vi "Measure vs B2D.vi"() -> ()   [LabVIEW 2009]
doc: "This VI is an example operator panel.\n\nThe VI contains a table for the field values that may be configured manually, or loaded by checking the \"Prompt for File\" box. The data file should contain 3 columns of data, with each column delimited by a tab character.\n\nBefore the VI is executed, set the desired field units and coordinate system. Once the VI is started, follow the directions in the STATUS indicator to operate. Once a field value is achieved, it will be held indefinitely with no user intervention.\n\nThe present field is displayed in the selected units and coordinate system. The present field is queried once per second.\n\nIf a field point is specified that is outside the limits for the magnet, the VI will abort execution."
uses:
  <vilib>/Utility/file.llb/Read From Spreadsheet File (DBL).vi
panel:
  in  "X Axis":enum16{"B", "phi"}(ring)
  in  "Y Axis":T1(ring)=enum."LI 1 Vx"
  out "measured data":dbl[][](array[numeric])
  out "XY Graph":T2(graph)
  in  "Notes:":string caption="Notizen:"
  out "Messfile Refnum":refnum<file>
  in  "Measurement File":path=path "D:/UserData/Matthias/Test/test.txt"
  in  "Sample name:":string
  in  "HP 1":bool
  in  "GPIB HP":string="8"
  in  "LI 4":bool
  in  "GPIB L 4":string="8"
  in  "LI 3":bool
  in  "GPIB L 3":string="8"
  in  "LI 2":bool
  in  "GPIB L 2":string="8"
  in  "LI 1":bool=TRUE
  in  "GPIB L 1":string="8"
  out "Number of lines":i32=2
  in  "Operation":u16(ring) items=["Stepwise", "Continous"]
  out "Ramp Rate along Vector (T/min)":dbl=0.17799999999999996 format="%.3f"
  out "Current Ramp Rate Z (T/min)":dbl=0.17799999911017794 format="%.3f"
  out "Current Ramp Rate Y (T/min)":dbl=1.7798220089008895e-05 format="%.3f"
  in  "User defined Ramp Rate (T/min)":bool=TRUE
  in  "User defined Ramp Rate (T/min)":dbl=0.178 format="%.3f"
  in  "Z-Axis Communications Config":T3={"GPIB address"=22, "GPIB bus"=1, "connection ID"=refnum, "IP"="111.111.111.1", "Active Comm Interface"=0, "Serial Port"="", "Programmer Type"=0} {"Programmer Type" items=["Model 430", "Model 420"]; "Active Comm Interface" items=["TCP/IP (Model 430 Only)", "RS232", "IEEE488"]}
  in  "Max Ramp Rate - Y Axis (A/s)":dbl=0.065 format="%.3f"
  in  "Max Ramp Rate - Z Axis (A/s)":dbl=0.203 format="%.3f"
  in  "Magnitude Limit (kG)":dbl=45.1 format="%.3f"
  in  "Y-Axis Communications Config":T3={"GPIB address"=22, "GPIB bus"=1, "connection ID"=refnum, "IP"="111.111.111.2", "Active Comm Interface"=0, "Serial Port"="", "Programmer Type"=0} {"Programmer Type" items=["Model 430", "Model 420"]; "Active Comm Interface" items=["TCP/IP (Model 430 Only)", "RS232", "IEEE488"]}
  out "Cartesian Display (T)":T4={"Y-Axis Field (T)"=-0.0, "Z-Axis Field (T)"=1e-05} {"Z-Axis Field (T)" format="%.3f"; "Y-Axis Field (T)" format="%.3f"}
  in  "Starting index":i32
  in  "Normal color":u32(colorbox)=11711154
  in  "Highlight color":u32(colorbox)=16711680
  out "?":string="American Magnetics, Inc."
  in  "Prompt for File?":bool
  out "Continue Execution?":bool=TRUE
  out "error out":T5
  in  "error in":T5
  out "STATUS":string="Holding at current vector. Set Ramping Mode to NEXT VECTOR to continue."
  in  "Ramping Control":u16(ring)=2 items=["NEXT VECTOR", "RAMPING", "HOLDING", "PAUSE", "ZERO"]
  out "Cartesian Display (kG)":T6 {"Z-Axis Field (kG)" format="%.3f"; "Y-Axis Field (kG)" format="%.3f"}
  in  "Field Values":string[][](table)=[["0", "0.1"], ["0", "0"]]
  out "Switch Heaters":bool=TRUE
  out "Polar Display (T)":T7={"q (degrees)"=90.0, "Field Magnitude (T)"=2e-05} {"Field Magnitude (T)" format="%.3f"; "q (degrees)" format="%.3f"}
  out "Polar Display (kG)":T8 {"Field Magnitude (kG)" format="%.3f"; "q (degrees)" format="%.3f"}
  in  "Coordinate System":u16(ring) items=["Cartesian", "Polar"]
  in  "Magnetic Field Units":u16(ring)=1 items=["kG", "Tesla"]
  # "Measurement Display"
  # "Measurement Settings"
  # "Magnet Settings"
  # "Devices"
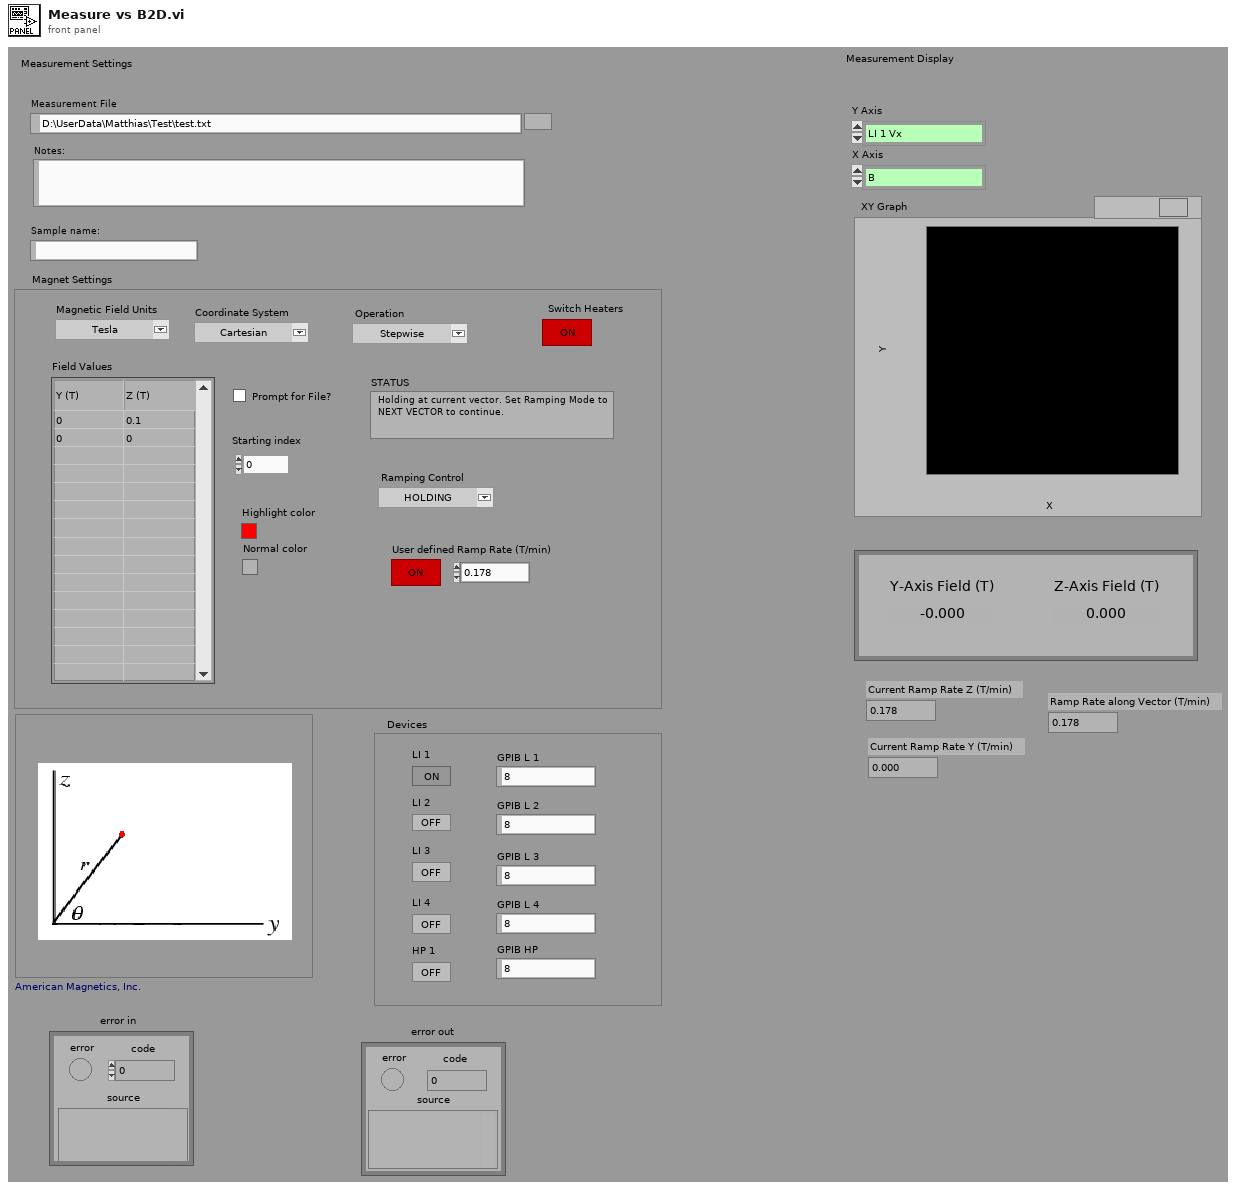
[diagram p1: front panel]
types:
  T1 = enum16{"B", "phi", "LI 1 Vx", "LI 1 phase", "LI 2 Vx", "LI 2 phase", "LI 3 Vx", "LI 3 phase", "LI 4 Vx", "LI 4 phase", "HP (V)"}
  T2 = cluster{"measured data":dbl[], "measured data":dbl[]}
  T3 = cluster{"GPIB address":i16, "GPIB bus":i16, "connection ID":refnum<k5>, "IP":string, "Active Comm Interface":u16, "Serial Port":refnum<visa-resource-name>, "Programmer Type":u16}
  T4 = cluster{"Y-Axis Field (T)":dbl, "Z-Axis Field (T)":dbl}
  T5 = cluster{"error":bool, "code":i32, "source":string}
  T6 = cluster{"Y-Axis Field (kG)":dbl, "Z-Axis Field (kG)":dbl}
  T7 = cluster{"q (degrees)":dbl, "Field Magnitude (T)":dbl}
  T8 = cluster{"q (degrees)":dbl, "Field Magnitude (kG)":dbl}
  T9 = enum16{"", "RAMPING", "HOLDING", "PAUSED", "MANUAL UP", "MANUAL DOWN", "ZEROING CURRENT", "QUENCH DETECTED", "HEATING SWITCH"}
  T10 = enum16{"", "RAMPING", "HOLDING", "PAUSED", "MANUAL UP", "MANUAL DOWN", "ZEROING CURRENT", "QUENCH DETECTED", "HEATING SWITCH", "AT ZER0", "COOLING SWITCH"}
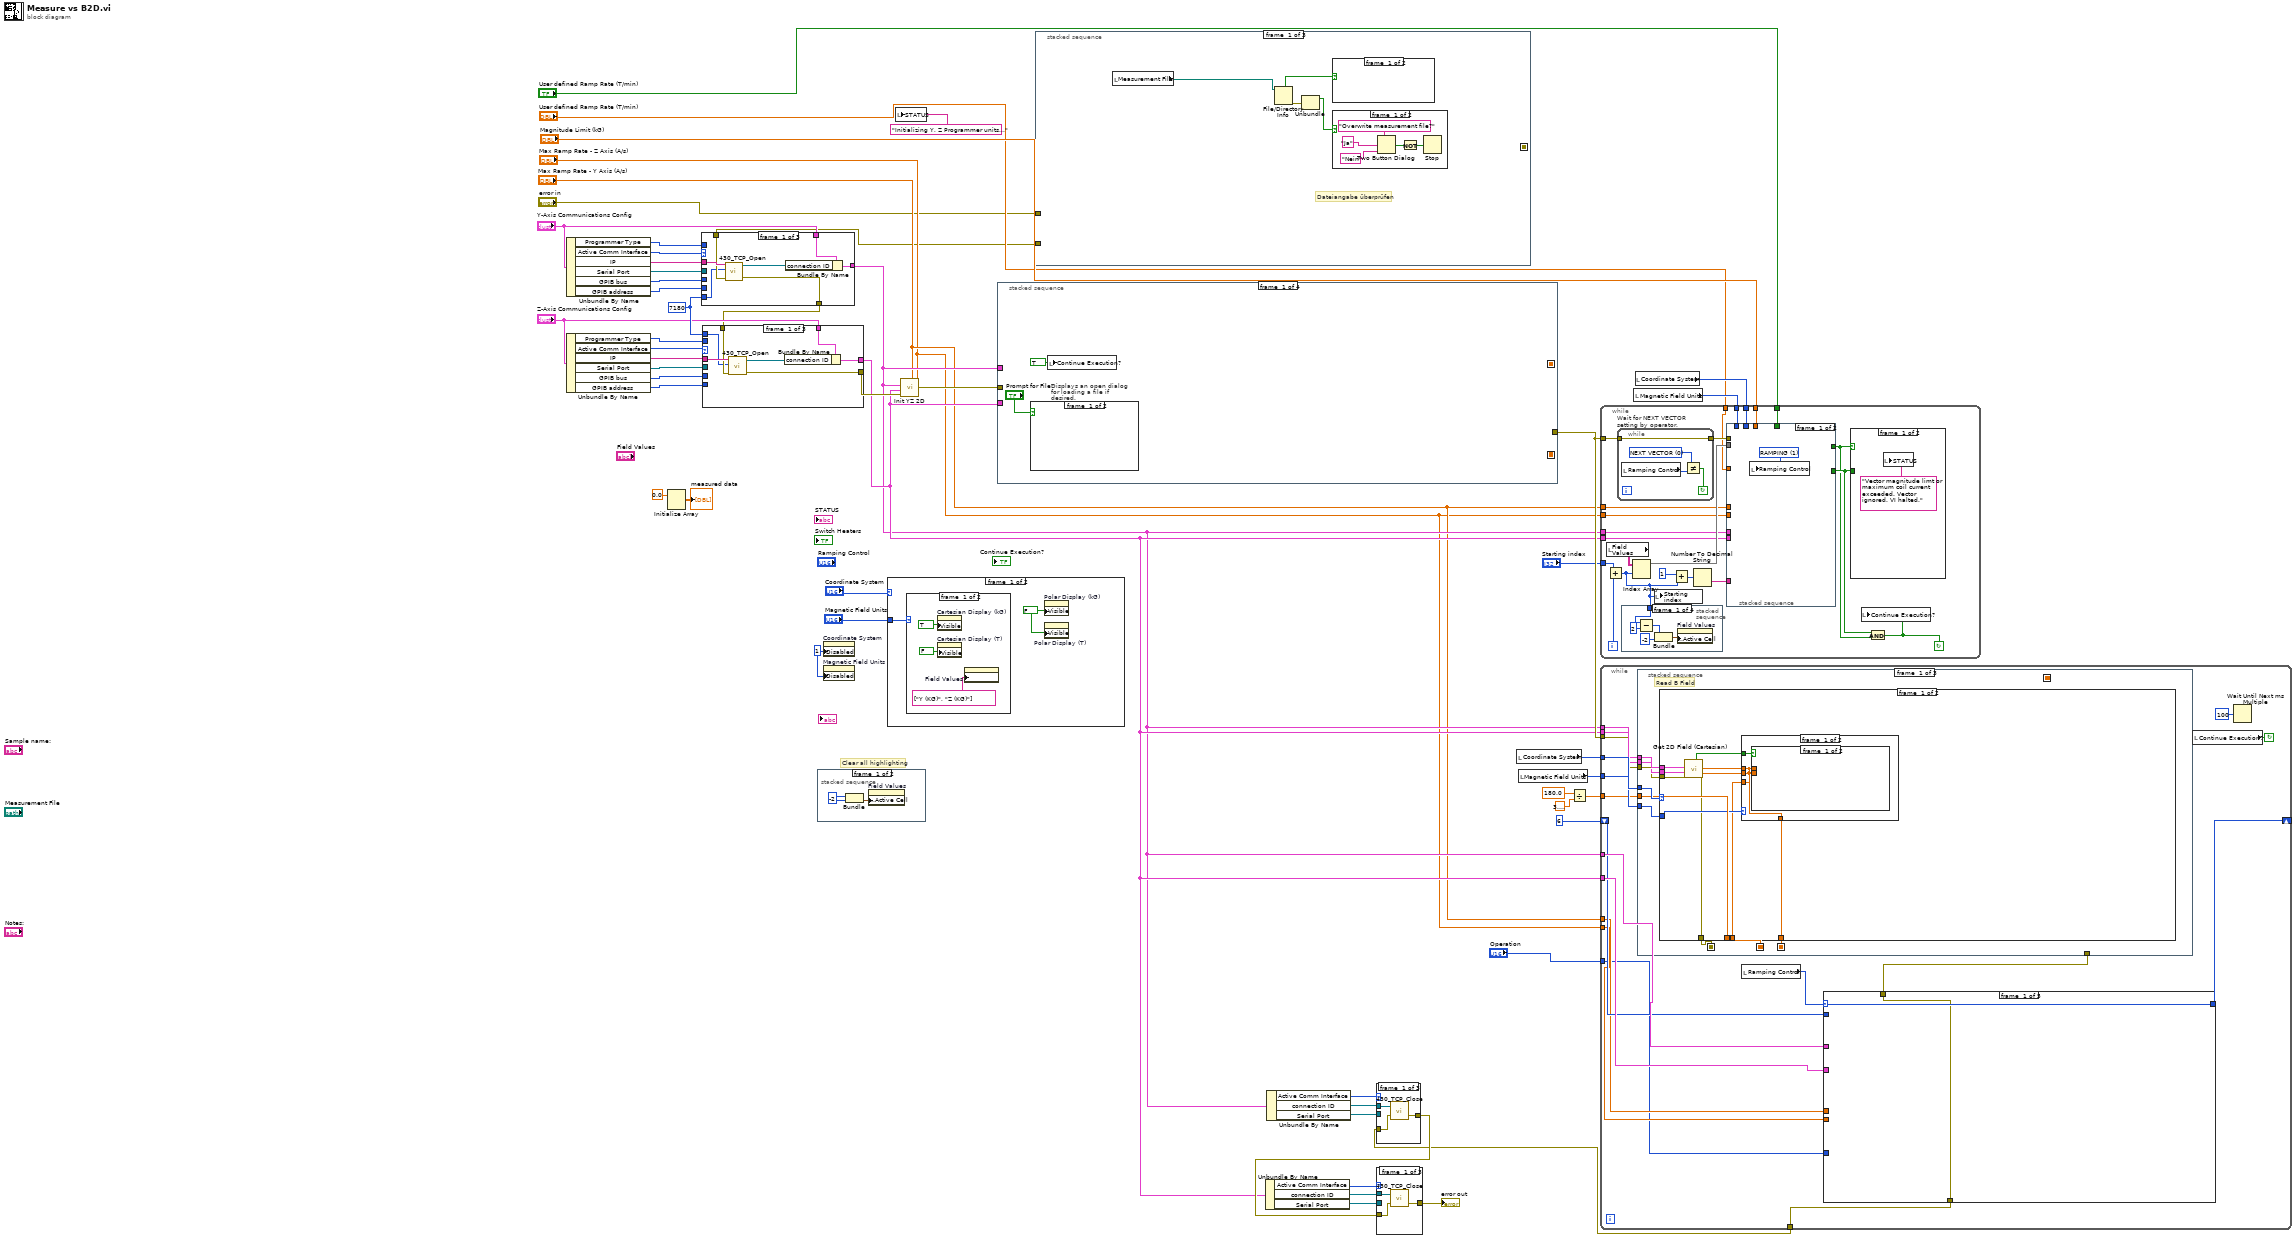
[diagram p0: block diagram]
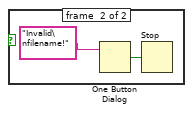
[diagram p3: hidden frame]
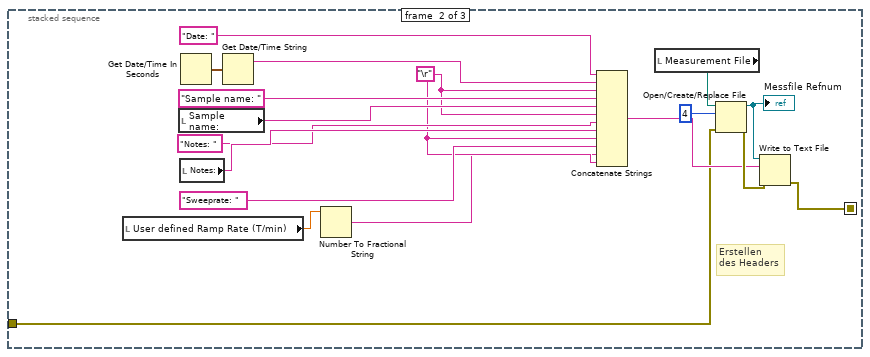
[diagram p4: hidden frame]
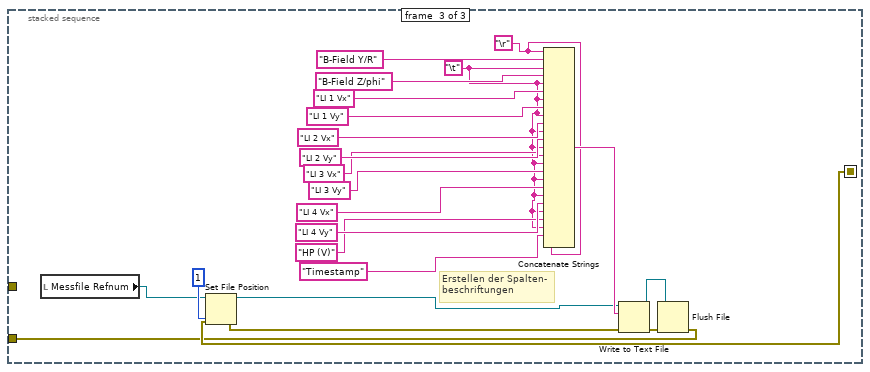
[diagram p5: hidden frame]
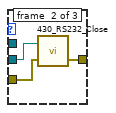
[diagram p6: hidden frame]
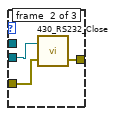
[diagram p8: hidden frame]
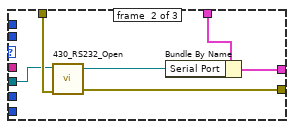
[diagram p10: hidden frame]
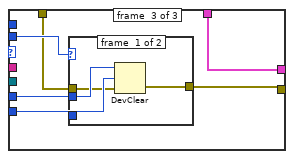
[diagram p11: hidden frame]
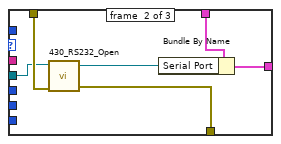
[diagram p13: hidden frame]
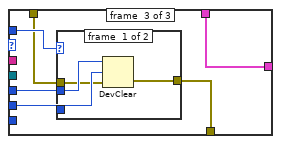
[diagram p14: hidden frame]
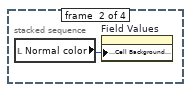
[diagram p16: hidden frame]
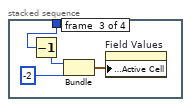
[diagram p17: hidden frame]
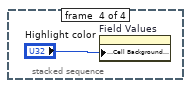
[diagram p18: hidden frame]
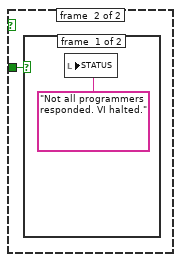
[diagram p19: hidden frame]
diagram:
  w38 = 7180 ("TCP Port")
  w51 = u8 1 ("Write Attribute")
  # "Clear all highlighting"
  n1 = Unbundle By Name("Z-Axis Communications Config") -> ("Programmer Type"=w14:u16, "Active Comm Interface"=w37:u16, "IP"=w34:string, "Serial Port"=w33:refnum<visa-resource-name>, "GPIB bus"=w13:i16, "GPIB address"=w12:i16)
  n2 = Unbundle By Name("Y-Axis Communications Config") -> ("Programmer Type"=w8:u16, "Active Comm Interface"=w36:u16, "IP"=w35:string, "Serial Port"=w32:refnum<visa-resource-name>, "GPIB bus"=w9:i16, "GPIB address"=w10:i16)
  n3 = Initialize Array(0.0 ("element")) -> (→"measured data":dbl[][])  [unwired: 2 in]
  n4 = stacked-sequence {
    frame #0 {
      w54 = -2
      n5 = Bundle(w54, w54) -> (w55:cluster{i32, i32})  [unwired: 1 in]
      n6 = property on="Field Values" class="Tbl (strict)"("Active Cell:Active Cell"=w55) -> ()  [unwired: 2 in, 2 out]
    }
    frame #1 {
      n7 = property on="Field Values" class="Tbl (strict)"("Active Cell:Cell Background Color"="Normal color") -> ()  [unwired: 2 in, 2 out]
    }
  }
  n8 = property on="Coordinate System" class="Ring (strict)"("Disabled"=w51) -> ()  [unwired: 2 in, 2 out]
  n9 = property on="Magnetic Field Units" class="Ring (strict)"("Disabled"=w51) -> ()  [unwired: 2 in, 2 out]
  n10 = case shown="1" "Coordinate System" {
    tunnel: "Magnetic Field Units" -> [w58 w66]
    frame #0 {
      w57 = FALSE ("Write Attribute")
      (unwired) FALSE ("Write Attribute")
      (unwired) TRUE ("Write Attribute")
      n11 = case shown="0, Default" w58 {
        frame #0 {
          n12 = property on="Cartesian Display (kG)" class="Cluster (strict)"("Visible"=TRUE ("Write Attribute")) -> ()  [unwired: 2 in, 2 out]
          n13 = property on="Cartesian Display (T)" class="Cluster (strict)"("Visible"=FALSE ("Write Attribute")) -> ()  [unwired: 2 in, 2 out]
          n14 = property on="Field Values" class="Tbl (strict)"("Column Header Strings[]"=string[] ["Y (KG)", "Z (KG)"] ("Write Attribute")) -> ()  [unwired: 2 in, 2 out]
        }
        frame #1 {
          n15 = property on="Cartesian Display (kG)" class="Cluster (strict)"("Visible"=FALSE ("Write Attribute")) -> ()  [unwired: 2 in, 2 out]
          n16 = property on="Cartesian Display (T)" class="Cluster (strict)"("Visible"=TRUE ("Write Attribute")) -> ()  [unwired: 2 in, 2 out]
          n17 = property on="Field Values" class="Tbl (strict)"("Column Header Strings[]"=string[] ["Y (T)", "Z (T)"] ("Write Attribute")) -> ()  [unwired: 2 in, 2 out]
        }
      }
      n18 = property on="Polar Display (kG)" class="Clust (strict)"("Visible"=w57) -> ()  [unwired: 2 in, 2 out]
      n19 = property on="Polar Display (T)" class="Clust (strict)"("Visible"=w57) -> ()  [unwired: 2 in, 2 out]
    }
    frame #1 {
      (unwired) FALSE ("Write Attribute")
      (unwired) TRUE ("Write Attribute")
      w65 = FALSE ("Write Attribute")
      n20 = case shown="1" w66 {
        frame #0 {
          n21 = property on="Polar Display (kG)" class="Clust (strict)"("Visible"=TRUE ("Write Attribute")) -> ()  [unwired: 2 in, 2 out]
          n22 = property on="Polar Display (T)" class="Clust (strict)"("Visible"=FALSE ("Write Attribute")) -> ()  [unwired: 2 in, 2 out]
          n23 = property on="Field Values" class="Tbl (strict)"("Column Header Strings[]"=string[] ["Mag. r (KG)", "Theta (deg)"] ("Write Attribute")) -> ()  [unwired: 2 in, 2 out]
        }
        frame #1 {
          n24 = property on="Polar Display (kG)" class="Clust (strict)"("Visible"=FALSE ("Write Attribute")) -> ()  [unwired: 2 in, 2 out]
          n25 = property on="Polar Display (T)" class="Clust (strict)"("Visible"=TRUE ("Write Attribute")) -> ()  [unwired: 2 in, 2 out]
          n26 = property on="Field Values" class="Tbl (strict)"("Column Header Strings[]"=string[] ["Mag. r (T)", "Theta (deg)"] ("Write Attribute")) -> ()  [unwired: 2 in, 2 out]
        }
      }
      n27 = property on="Cartesian Display (kG)" class="Cluster (strict)"("Visible"=w65) -> ()  [unwired: 2 in, 2 out]
      n28 = property on="Cartesian Display (T)" class="Cluster (strict)"("Visible"=w65) -> ()  [unwired: 2 in, 2 out]
    }
  }
  n29 = local write "STATUS"("Initializing Y, Z Programmer units..." ("STATUS")) -> ()
  n30 = stacked-sequence {
    seq-local: [_ w84 _] -> [_ _ w103]
    tunnel: "error in" -> [_ w85 _]
    tunnel: [_ _ w102] -> w3
    frame #0 {
      # "Dateiangabe überprüfen"
      n31 = local read "Measurement File"() -> (w76:path)
      n32 = File/Directory Info(path=w76) -> (directory=w74:bool, error out=w75:errorcluster)  [unwired: 1 in, 5 out]
      n33 = Unbundle(w75) -> ("status"=w73:bool)  [unwired: 2 out]
      n34 = case shown="False" w74 {
        frame #0 {
        }
        frame #1 {
          n35 = One Button Dialog(message="Invalid\nfilename!") -> (true=w82:bool)  [unwired: 1 in]
          n36 = Stop(stop? (T)=w82) -> ()
        }
      }
      n37 = case shown="False" w73 {
        frame #0 {
          n38 = Two Button Dialog(message="Overwrite measurement file?", 1:"Nein", 2:"Ja") -> (T button?=w78:bool)
          n39 = Not(x=w78) -> (.not. x?=w77:bool)
          n40 = Stop(stop? (T)=w77) -> ()
        }
        frame #1 {
        }
      }
    }
    frame #1 {
      w88 = "\r"
      # "Erstellen\ndes Headers"
      n41 = local read "User defined Ramp Rate (T/min)"() -> (w87:dbl)
      n42 = local read "Sample name:"() -> (w94:string)
      n43 = local read "Notes:"() -> (w96:string)
      n44 = Get Date/Time In Seconds() -> (seconds since 1Jan1904=w90:timestamp)
      n45 = Get Date/Time String(seconds (now)=w90) -> (date string=w92:string)  [unwired: 2 in, 1 out]
      n46 = Number To Fractional String(number=w87) -> (F-format string=w86:string)  [unwired: 3 in]
      n47 = Concatenate Strings("Date: ", w92, w88, "Sample name: ", w94, w88, "Notes: ", w96, w88, "Sweeprate: ", w86, w88) -> (w100:string)
      n48 = local read "Measurement File"() -> (w97:path)
      n49 = Open/Create/Replace File(file path (use dialog)=w97, error in=w85, operation (0:open)=4) -> (refnum out=w99:refnum<file>, error out=w101:errorcluster)  [unwired: 3 in, 1 out]
      "Messfile Refnum" <- w99
      n50 = Write to Text File(file (use dialog)=w99, text=w100, error in=w101) -> (error out=w84:errorcluster)  [unwired: 1 in, 2 out]
    }
    frame #2 {
      w106 = "\t"
      w104 = "\r"
      # "Erstellen der Spalten-\nbeschriftungen"
      n51 = local read "Messfile Refnum"() -> (w113:refnum<file>)
      n52 = Set File Position(refnum=w113, from (0:start)=1, error in=w103) -> (refnum out=w119:refnum<file>, error out=w121:errorcluster)  [unwired: 1 in]
      n53 = Concatenate Strings(w104, "B-Field Y/R", w106, "B-Field Z/phi", w106, "LI 1 Vx", w106, "LI 1 Vy", w106, "LI 2 Vx", w106, "LI 2 Vy", w106, "LI 3 Vx", w106, "LI 3 Vy", w106, "LI 4 Vx", w106, "LI 4 Vy", w106, "HP (V)", w106, "Timestamp", w104) -> (w120:string)
      n54 = Write to Text File(file (use dialog)=w119, text=w120, error in=w121) -> (refnum out=w123:refnum<file>, error out=w122:errorcluster)  [unwired: 1 in, 1 out]
      n55 = Flush File(refnum=w123, error in=w122) -> (error out=w102:errorcluster)  [unwired: 1 out]
    }
  }
  n56 = case shown="2" w36 {
    tunnel: w35 -> [w131 _ _]
    tunnel: w3 -> [w130 w137 w139]
    tunnel: "Y-Axis Communications Config" -> [w129 w132 w143]
    tunnel: [w127 w135 w143] -> w21
    tunnel: [w126 w136 w138] -> w11
    tunnel: w38 -> [w125 _ _]
    tunnel: w32 -> [_ w133 _]
    tunnel: w10 -> [_ _ w142]
    tunnel: w9 -> [_ _ w141]
    tunnel: w8 -> [_ _ w140]
    frame #0 {
      n57 = call <userlib>:"430_TCP_Open.vi"("IP Address"=w131, "TCP Port"=w125, "error in (no error)"=w130) -> ("connection ID"=w128:refnum<k5>, "error out"=w126:errorcluster)  [unwired: 3 in, 1 out]
      n58 = Bundle By Name(cluster=w129, "connection ID"=w128) -> (w127:T3)
    }
    frame #1 {
      n59 = call <userlib>:"430_RS232_Open.vi"("VISA resource name"=w133, "error in (no error)"=w137) -> ("VISA resource name out"=w134:refnum<visa-resource-name>, "error out"=w136:errorcluster)  [unwired: 5 in]
      n60 = Bundle By Name(cluster=w132, "Serial Port"=w134) -> (w135:T3)
    }
    frame #2 {
      n61 = case shown="0, Default" w140 {
        tunnel: w141 -> [w147 _]
        tunnel: w142 -> [w146 _]
        tunnel: w139 -> [w145 w148]
        tunnel: [w144 w148] -> w138
        frame #0 {
          n62 = DevClear(2:w145, 3:w146, 4:w147) -> (0:w144:errorcluster)  [unwired: 1 out]
        }
        frame #1 {
        }
      }
    }
  }
  n63 = case shown="2" w37 {
    tunnel: w34 -> [w155 _ _]
    tunnel: w11 -> [w154 w161 w163]
    tunnel: [w153 w160 w162] -> w31
    tunnel: "Z-Axis Communications Config" -> [w152 w158 w167]
    tunnel: [w150 w159 w167] -> w22
    tunnel: w38 -> [w149 _ _]
    tunnel: w33 -> [_ w156 _]
    tunnel: w14 -> [_ _ w166]
    tunnel: w13 -> [_ _ w165]
    tunnel: w12 -> [_ _ w164]
    frame #0 {
      n64 = call <userlib>:"430_TCP_Open.vi"("IP Address"=w155, "TCP Port"=w149, "error in (no error)"=w154) -> ("connection ID"=w151:refnum<k5>, "error out"=w153:errorcluster)  [unwired: 3 in, 1 out]
      n65 = Bundle By Name(cluster=w152, "connection ID"=w151) -> (w150:T3)
    }
    frame #1 {
      n66 = call <userlib>:"430_RS232_Open.vi"("VISA resource name"=w156, "error in (no error)"=w161) -> ("VISA resource name out"=w157:refnum<visa-resource-name>, "error out"=w160:errorcluster)  [unwired: 5 in]
      n67 = Bundle By Name(cluster=w158, "Serial Port"=w157) -> (w159:T3)
    }
    frame #2 {
      n68 = case shown="0, Default" w166 {
        tunnel: w165 -> [w171 _]
        tunnel: w164 -> [w170 _]
        tunnel: w163 -> [w169 w172]
        tunnel: [w168 w172] -> w162
        frame #0 {
          n69 = DevClear(2:w169, 3:w170, 4:w171) -> (0:w168:errorcluster)  [unwired: 1 out]
        }
        frame #1 {
        }
      }
    }
  }
  n70 = call <userlib>:"Init YZ 2D.vi"("Max Ramp Rate Z-axis"="Max Ramp Rate - Z Axis (A/s)", "Max Ramp Rate Y-axis"="Max Ramp Rate - Y Axis (A/s)", "error in"=w31, "Z-Axis Communications Config"=w22, "Y-Axis Communications Config"=w21) -> ("error out"=w49:T5)  [unwired: 5 in]
  n71 = stacked-sequence {
    seq-local: [_ w180 _ _] -> [_ _ w227 _]
    seq-local: [_ w179 _ _] -> [_ _ w226 _]
    tunnel: w22 -> [_ w182 _ _]
    tunnel: w49 -> [_ w183 _ _]
    tunnel: [_ w178 _ _] -> w45
    tunnel: w21 -> [_ w181 _ _]
    frame #0 {
      n72 = case "Displays an open dialog for loading a file if desired." shown="True" "Prompt for File?" {
        frame #0 {
        }
        frame #1 {
          n73 = call-poly <vilib>:"Read From Spreadsheet File.vi"() -> ("all rows"=w177:dbl[][])  [unwired: 7 in, 4 out]
          n74 = Number To Fractional String(number=w177, precision (6)=i16 4) -> (F-format string=w176:string[][])  [unwired: 2 in]
          n75 = local write "Field Values"(w176) -> ()
        }
      }
      n76 = local write "Continue Execution?"(TRUE ("Continue Execution?")) -> ()
    }
    frame #1 {
      w191 = u16 3 items=["NEXT VECTOR", "RAMPING", "HOLDING", "PAUSE", "ZERO"] ("Ramping Control")
      n77 = call <userlib>:"Get Switch Present.vi"("error in"=w183, "Communications Config"=w181) -> ("error out"=w187:T5, "Switch Present?"=w188:bool)
      n78 = case shown="True" w188 {
        tunnel: w187 -> [w209 w218]
        tunnel: w181 -> [_ w211]
        tunnel: [0.0 w215] -> w179
        tunnel: [w209 w217] -> w186
        frame #0 {
        }
        frame #1 {
          n79 = call <userlib>:"Get Switch Heater Time.vi"("error in"=w218, "Communications Config"=w211) -> ("error out"=w214:T5, "Switch Heating Time (secs)"=w216:dbl)
          n80 = call <userlib>:"Get Switch Heater.vi"("error in"=w214, "Communications Config"=w211) -> ("error out"=w213:T5, "Switch Heater Indicator"=w212:bool)
          n81 = case shown="False" w212 {
            tunnel: [w223 w224] -> w217
            tunnel: w216 -> [w221 _]
            tunnel: [w221 0.0] -> w215
            tunnel: w213 -> [w219 w224]
            tunnel: w211 -> [w220 _]
            frame #0 {
              n82 = call <userlib>:"Set Switch Heater.vi"("error in"=w219, "Switch Heater Control"=TRUE, "Communications Config"=w220) -> ("error out"=w223:T5)
            }
            frame #1 {
            }
          }
        }
      }
      n83 = call <userlib>:"Get Switch Present.vi"("error in"=w186, "Communications Config"=w182) -> ("error out"=w184:T5, "Switch Present?"=w185:bool)
      n84 = case shown="True" w185 {
        tunnel: w184 -> [w192 w201]
        tunnel: w182 -> [_ w194]
        tunnel: [0.0 w198] -> w180
        tunnel: [w192 w200] -> w178
        frame #0 {
        }
        frame #1 {
          n85 = call <userlib>:"Get Switch Heater Time.vi"("error in"=w201, "Communications Config"=w194) -> ("error out"=w197:T5, "Switch Heating Time (secs)"=w199:dbl)
          n86 = call <userlib>:"Get Switch Heater.vi"("error in"=w197, "Communications Config"=w194) -> ("error out"=w196:T5, "Switch Heater Indicator"=w195:bool)
          n87 = case shown="False" w195 {
            tunnel: [w202 w207] -> w200
            tunnel: w199 -> [w205 _]
            tunnel: [w205 0.0] -> w198
            tunnel: w196 -> [w203 w207]
            tunnel: w194 -> [w204 _]
            frame #0 {
              n88 = call <userlib>:"Set Switch Heater.vi"("error in"=w203, "Switch Heater Control"=TRUE, "Communications Config"=w204) -> ("error out"=w202:T5)
            }
            frame #1 {
            }
          }
        }
      }
      n89 = local write "Ramping Control"(w191) -> ()
      n90 = local write "Switch Heaters"(TRUE ("Switch Heater Control")) -> ()
      n91 = property on="Switch Heaters" class="Boolean (strict)"("Disabled"=u8 1 ("Write Attribute")) -> ()  [unwired: 2 in, 2 out]
    }
    frame #2 {
      n92 = Max & Min(x=w227, y=w226) -> (max(x,y)=w228:dbl)  [unwired: 1 out]
      n93 = local write "STATUS"("Heating switches..." ("STATUS")) -> ()
      n94 = Add(x=w228, y=2) -> (x+y=w232:dbl)
      n95 = property on="Ramping Control" class="Ring (strict)"("Disabled"=u8 1 ("Write Attribute")) -> ()  [unwired: 2 in, 2 out]
      n96 = Multiply(x=w232, y=1000) -> (x*y=w231:dbl)
      n97 = Wait (ms)(milliseconds to wait=w231) -> ()  [unwired: 1 out]
    }
    frame #3 {
      n98 = property on="Ramping Control" class="Ring (strict)"("Disabled"=u8 0 ("Write Attribute")) -> ()  [unwired: 2 in, 2 out]
      n99 = local write "STATUS"("Ready to ramp to first vector. Set Ramping Mode to NEXT VECTOR to begin." ("STATUS")) -> ()
      n100 = local read "Field Values"() -> (w237:string[][])
      n101 = Array Size(array=w237) -> (size(s)=w236:i32[])
      n102 = Index Array(array=w236, index=0) -> (element=→"Number of lines":i32)
    }
  }
  n103 = Unbundle By Name(w22) -> ("Active Comm Interface"=w28:u16, "connection ID"=w27:refnum<k5>, "Serial Port"=w26:refnum<visa-resource-name>)
  n104 = Unbundle By Name(w21) -> ("Active Comm Interface"=w29:u16, "connection ID"=w25:refnum<k5>, "Serial Port"=w24:refnum<visa-resource-name>)
  n105 = local read "Coordinate System"() -> (w46:u16)
  n106 = local read "Magnetic Field Units"() -> (w44:u16)
  n107 = Divide(x=180.0, y=3.141592653589793) -> (x/y=w41:dbl)
  n108 = while {
    shift-left: u16 6 ("Ramping Control") -> [w245]
    shift-right: [w246] -> _
    tunnel: [w248] -> w23
    tunnel: w22 -> [w249]
    tunnel: w21 -> [w250]
    tunnel: w41 -> [w252]
    tunnel: w44 -> [w253]
    tunnel: w45 -> [w254]
    tunnel: w22 -> [w255]
    tunnel: w21 -> [w256]
    tunnel: w46 -> [w257]
    tunnel: "Max Ramp Rate - Y Axis (A/s)" -> [w244]
    tunnel: "Max Ramp Rate - Z Axis (A/s)" -> [w243]
    tunnel: "Operation" -> [w242]
    stop <- w247 continue-if-true
    n109 = stacked-sequence {
      seq-local: [w261 _ _] -> [_ w349 _]
      seq-local: [w260 _ _] -> [_ w343 _]
      seq-local: [w259 _ _] -> [_ w344 _]
      seq-local: [_ w330 _] -> [_ _ w410]
      tunnel: w257 -> [w267 _ w408]
      tunnel: w256 -> [w266 _ _]
      tunnel: w255 -> [w265 _ _]
      tunnel: w254 -> [w264 _ _]
      tunnel: w253 -> [w263 _ _]
      tunnel: w252 -> [w262 _ _]
      tunnel: [_ w345 _] -> w241
      frame #0 {
        # "Read B Field"
        n110 = case shown="1" w267 {
          tunnel: w266 -> [w277 w300]
          tunnel: w265 -> [w276 w299]
          tunnel: w264 -> [w275 w298]
          tunnel: w263 -> [w274 w297]
          tunnel: w262 -> [_ w296]
          tunnel: [w270 w295] -> w261
          tunnel: [w269 w293] -> w260
          tunnel: [w268 w294] -> w259
          frame #0 {
            n111 = call <userlib>:"Get 2D Field (Cartesian).vi"("Y-Axis Communications Config"=w277, "Z-Axis Communications Config"=w276, "error in"=w275) -> ("All Instruments Responded?"=w271:bool, "Y-Axis Field (kG)"=w273:dbl, "Z-Axis Field (kG)"=w272:dbl, "error out"=w270:T5)  [unwired: 2 in]
            n112 = case shown="0, Default" w274 {
              tunnel: w273 -> [w278 w286]
              tunnel: w272 -> [w279 w287]
              tunnel: w271 -> [w280 w289]
              tunnel: [w279 w285] -> w269
              tunnel: [w278 w284] -> w268
              frame #0 {
                n113 = case shown="True" w280 {
                  tunnel: w278 -> [_ w282]
                  tunnel: w279 -> [_ w281]
                  frame #0 {
                  }
                  frame #1 {
                    n114 = Bundle("Y-Axis Field (kG)"=w282, "Z-Axis Field (kG)"=w281) -> (→"Cartesian Display (kG)":T6)  [unwired: 1 in]
                  }
                }
              }
              frame #1 {
                w288 = 0.1 ("y")
                n115 = Multiply(x=w286, y=w288) -> (x*y=w284:dbl)
                n116 = Multiply(x=w287, y=w288) -> (x*y=w285:dbl)
                n117 = case shown="False" w289 {
                  tunnel: w284 -> [_ w292]
                  tunnel: w285 -> [_ w291]
                  frame #0 {
                  }
                  frame #1 {
                    n118 = Bundle(w292, w291) -> (→"Cartesian Display (T)":cluster{dbl, dbl})  [unwired: 1 in]
                  }
                }
              }
            }
          }
          frame #1 {
            n119 = stacked-sequence {
              tunnel: w300 -> [w311]
              tunnel: w299 -> [w310]
              tunnel: w298 -> [w309]
              tunnel: w297 -> [w308]
              tunnel: w296 -> [w305]
              tunnel: [w303] -> w295
              tunnel: [w302] -> w294
              tunnel: [w301] -> w293
              frame #0 {
                # "Field"
                n120 = call <userlib>:"Get 2D Field (Polar).vi"("Y-Axis Communications Config"=w311, "Z-Axis Communications Config"=w310, "error in"=w309) -> ("All Instruments Responded?"=w304:bool, "Radial (r) Field (kG)"=w307:dbl, "q (radians)"=w306:dbl, "error out"=w303:T5)  [unwired: 2 in]
                n121 = case shown="0, Default" w308 {
                  tunnel: w307 -> [w313 w325]
                  tunnel: w306 -> [w315 w324]
                  tunnel: w305 -> [w314 w323]
                  tunnel: w304 -> [w316 w322]
                  tunnel: [w313 w320] -> w302
                  tunnel: [w312 w321] -> w301
                  frame #0 {
                    n122 = Multiply(x=w315, y=w314) -> (x*y=w312:dbl)
                    n123 = case shown="False" w316 {
                      tunnel: w313 -> [_ w317]
                      tunnel: w312 -> [_ w318]
                      frame #0 {
                      }
                      frame #1 {
                        n124 = Bundle(w318, "Radial (r) Field (kG)"=w317) -> (→"Polar Display (kG)":cluster{dbl, "Radial (r) Field (kG)":dbl})  [unwired: 1 in]
                      }
                    }
                  }
                  frame #1 {
                    n125 = Multiply(x=w325, y=0.1) -> (x*y=w321:dbl)
                    n126 = Multiply(x=w324, y=w323) -> (x*y=w320:dbl)
                    n127 = case shown="True" w322 {
                      tunnel: w321 -> [_ w327]
                      tunnel: w320 -> [_ w328]
                      frame #0 {
                      }
                      frame #1 {
                        n128 = Bundle(w328, w327) -> (→"Polar Display (T)":cluster{dbl, dbl})  [unwired: 1 in]
                      }
                    }
                  }
                }
              }
            }
          }
        }
      }
      frame #1 {
        # "Zeile in Datei schreiben"
        # "Read and Save Devices"
        n129 = stacked-sequence {
          tunnel: [w354 _ _ _ _ _] -> w342
          tunnel: [w353 _ _ _ _ _] -> w341
          tunnel: [_ w367 _ _ _ _] -> w338
          tunnel: [_ w365 _ _ _ _] -> w337
          tunnel: [_ _ w377 _ _ _] -> w336
          tunnel: [_ _ w376 _ _ _] -> w335
          tunnel: [_ _ _ w388 _ _] -> w334
          tunnel: [_ _ _ w387 _ _] -> w333
          tunnel: [_ _ _ _ w398 _] -> w332
          tunnel: [_ _ _ _ _ w404] -> w331
          frame #0 {
            n130 = case shown="True" "LI 1" {
              tunnel: ["0" ("Antwort2") w361] -> w356
              tunnel: ["0" ("Antwort1") w360] -> w355
              frame #0 {
              }
              frame #1 {
                n131 = call "LI-Ansteuerung.vi"("Frage2"="OUTP? 4", "Frage1"="OUTP? 1", "address string"="GPIB L 1") -> ("Antwort2"=w361:string, "Antwort1"=w360:string)
              }
            }
            n132 = Fract/Exp String To Number(string=w356) -> (number=w353:dbl)  [unwired: 3 in, 1 out]
            n133 = Fract/Exp String To Number(string=w355) -> (number=w354:dbl)  [unwired: 3 in, 1 out]
          }
          frame #1 {
            n134 = case shown="False" "LI 2" {
              tunnel: [w370 w372] -> w366
              tunnel: [w370 w371] -> w368
              frame #0 {
                w370 = "0" ("Antwort1")
              }
              frame #1 {
                n135 = call "LI-Ansteuerung.vi"("Frage2"="OUTP? 4", "Frage1"="OUTP? 1", "address string"="GPIB L 2") -> ("Antwort2"=w372:string, "Antwort1"=w371:string)
              }
            }
            n136 = Fract/Exp String To Number(string=w366) -> (number=w365:dbl)  [unwired: 3 in, 1 out]
            n137 = Fract/Exp String To Number(string=w368) -> (number=w367:dbl)  [unwired: 3 in, 1 out]
          }
          frame #2 {
            n138 = case shown="False" "LI 3" {
              tunnel: [w381 w383] -> w378
              tunnel: [w381 w382] -> w379
              frame #0 {
                w381 = "0" ("Antwort1")
              }
              frame #1 {
                n139 = call "LI-Ansteuerung.vi"("Frage2"="OUTP? 4", "Frage1"="OUTP? 1", "address string"="GPIB L 3") -> ("Antwort2"=w383:string, "Antwort1"=w382:string)
              }
            }
            n140 = Fract/Exp String To Number(string=w379) -> (number=w377:dbl)  [unwired: 3 in, 1 out]
            n141 = Fract/Exp String To Number(string=w378) -> (number=w376:dbl)  [unwired: 3 in, 1 out]
          }
          frame #3 {
            n142 = case shown="True" "LI 4" {
              tunnel: [w392 w394] -> w389
              tunnel: [w392 w393] -> w390
              frame #0 {
                w392 = "0" ("Antwort1")
              }
              frame #1 {
                n143 = call "LI-Ansteuerung.vi"("Frage2"="OUTP? 4", "Frage1"="OUTP? 1", "address string"="GPIB L 4") -> ("Antwort2"=w394:string, "Antwort1"=w393:string)
              }
            }
            n144 = Fract/Exp String To Number(string=w389) -> (number=w387:dbl)  [unwired: 3 in, 1 out]
            n145 = Fract/Exp String To Number(string=w390) -> (number=w388:dbl)  [unwired: 3 in, 1 out]
          }
          frame #4 {
            n146 = case shown="True" "HP 1" {
              tunnel: [0.0 ("Voltage") w402] -> w398
              frame #0 {
              }
              frame #1 {
                n147 = call "HP-ReadVoltagev2.vi"("String"="meas:volt:dc? 100,0.0001", "HP-Mulitmeter\nGPIB Address"="GPIB HP") -> ("Voltage"=w402:dbl)  [unwired: 9 in]
              }
            }
          }
          frame #5 {
            n148 = Get Date/Time In Seconds() -> (seconds since 1Jan1904=w405:timestamp)
            n149 = To Double Precision Float(number=w405) -> (double precision float=w404:dbl)
          }
        }
        n150 = Build Array(w344, w343, w342, w341, w338, w337, w335, w336, w334, w333, w332, w331) -> (w330:dbl[])
        n151 = Array To Spreadsheet String(array=w330, 3:"%f" ("format string")) -> (spreadsheet string=w340:string)  [unwired: 1 in]
        n152 = local read "Messfile Refnum"() -> (w346:refnum<file>)
        n153 = Set File Position(refnum=w346, from (0:start)=1, error in=w349) -> (refnum out=w348:refnum<file>, error out=w350:errorcluster)  [unwired: 1 in]
        n154 = Write to Text File(file (use dialog)=w348, text=w340, error in=w350) -> (refnum out=w352:refnum<file>, error out=w351:errorcluster)  [unwired: 1 in, 1 out]
        n155 = Flush File(refnum=w352, error in=w351) -> (error out=w345:errorcluster)  [unwired: 1 out]
      }
      frame #2 {
        n156 = local read "measured data"() -> (w411:dbl[][])
        n157 = Insert Into Array(array=w411, new element=w410) -> (w409:dbl[][])  [unwired: 2 in]
        n158 = case shown="0, Default" w408 {
          tunnel: w409 -> [w427 w441]
          tunnel: "Y Axis" -> [w429 w440]
          tunnel: "X Axis" -> [w415 w439]
          frame #0 {
            n159 = Index Array(array=w427, index (col)=1 ("disabled index (col)")) -> (element=w422:dbl[])  [unwired: 1 in]
            n160 = Index Array(array=w427, index (col)=0 ("disabled index (col)")) -> (element=w421:dbl[])  [unwired: 1 in]
            n161 = Square(x=w422) -> (x^2=w424:dbl[])
            n162 = Square(x=w421) -> (x^2=w425:dbl[])
            n163 = Index Array(array=w427, index (col)=w429) -> (element=w414:dbl[])  [unwired: 1 in]
            n164 = Divide(x=w422, y=w421) -> (x/y=w420:dbl[])
            n165 = Add(x=w425, y=w424) -> (x+y=w423:dbl[])
            n166 = Tangent(1:w420) -> (0:w419:dbl[])
            n167 = Square Root(x=w423) -> (sqrt(x)=w412:dbl[])
            n168 = Divide(x=w419, y=3.141592653589793) -> (x/y=w417:dbl[])
            n169 = Multiply(x=w417, y=180) -> (x*y=w413:dbl[])
            n170 = case shown="\"B\", Default" w415 {
              tunnel: w414 -> [w432 w435]
              tunnel: w413 -> [_ w434]
              tunnel: w412 -> [w431 _]
              frame #0 {
                n171 = Bundle(w431, "measured data"=w432) -> (w430:cluster{dbl[], "measured data":dbl[]})  [unwired: 1 in]
                n172 = local write "XY Graph"(w430) -> ()
              }
              frame #1 {
                n173 = Bundle(w434, "measured data"=w435) -> (w433:cluster{dbl[], "measured data":dbl[]})  [unwired: 1 in]
                n174 = local write "XY Graph"(w433) -> ()
              }
            }
          }
          frame #1 {
            n175 = Index Array(array=w441, index (col)=w439) -> (element=w438:dbl[])  [unwired: 1 in]
            n176 = Index Array(array=w441, index (col)=w440) -> (element=w437:dbl[])  [unwired: 1 in]
            n177 = Bundle("measured data"=w438, "measured data"=w437) -> (w436:T2)  [unwired: 1 in]
            n178 = local write "XY Graph"(w436) -> ()
          }
        }
        n179 = local write "measured data"(w409) -> ()
      }
    }
    n180 = local read "Ramping Control"() -> (w251:u16)
    n181 = case shown="4" w251 {
      selector: w251 -> [w443 w456 w470 w474 w489]
      tunnel: w250 -> [_ w459 _ w477 w494]
      tunnel: w249 -> [_ w458 _ w476 w493]
      tunnel: [w442 w457 w469 w475 w492] -> w248
      tunnel: [w443 w456 w470 w474 w489] -> w246
      tunnel: w245 -> [_ _ _ w473 w491]
      tunnel: w244 -> [_ _ _ _ w488]
      tunnel: w243 -> [_ _ _ _ w487]
      tunnel: w242 -> [_ w448 _ _ _]
      tunnel: w241 -> [w442 w444 w469 w471 w486]
      frame #0 {
      }
      frame #1 {
        w451 = T9."HOLDING" ("y")
        n182 = local read "Number of lines"() -> (w445:i32)
        n183 = local read "Starting index"() -> (w447:i32)
        n184 = call <userlib>:"Get Ramping Mode.vi"("Communications Config"=w459, "error in"=w444) -> ("Ramping Mode"=w454:T10, "error out"=w455:T5)  [unwired: 1 out]
        n185 = call <userlib>:"Get Ramping Mode.vi"("Communications Config"=w458, "error in"=w455) -> ("Ramping Mode"=w453:T10, "error out"=w457:T5)  [unwired: 1 out]
        n186 = Less?(x=w447, y=w445) -> (x < y?=w446:bool)
        n187 = Equal?(x=w454, y=w451) -> (x = y?=w450:bool)
        n188 = Equal?(x=w453, y=w451) -> (x = y?=w449:bool)
        n189 = Compound Arithmetic op=AND(w450, w449) -> (w452:bool)
        n190 = case shown="True" w452 {
          tunnel: w448 -> [_ w461]
          tunnel: w446 -> [_ w460]
          frame #0 {
          }
          frame #1 {
            n191 = case shown="1" w461 {
              tunnel: w460 -> [_ w464]
              frame #0 {
                w463 = u16 2 items=["NEXT VECTOR", "RAMPING", "HOLDING", "PAUSE", "ZERO"] ("Ramping Control")
                n192 = local write "STATUS"("Holding at current vector. Set Ramping Mode to NEXT VECTOR to continue." ("STATUS")) -> ()
                n193 = local write "Ramping Control"(w463) -> ()
              }
              frame #1 {
                # "Go to NEXT VECTOR automatically"
                n194 = case shown="True" w464 {
                  frame #0 {
                    w466 = u16 2 items=["NEXT VECTOR", "RAMPING", "HOLDING", "PAUSE", "ZERO"] ("Ramping Control")
                    n195 = local write "STATUS"("Holding at current vector. Set Ramping Mode to NEXT VECTOR to continue." ("STATUS")) -> ()
                    n196 = local write "Ramping Control"(w466) -> ()
                  }
                  frame #1 {
                    w468 = u16 0 items=["NEXT VECTOR", "RAMPING", "HOLDING", "PAUSE", "ZERO"] ("Ramping Control")
                    n197 = local write "Ramping Control"(w468) -> ()
                    n198 = local write "STATUS"("Go to NEXT VECTOR" ("STATUS")) -> ()
                  }
                }
              }
            }
          }
        }
      }
      frame #2 {
      }
      frame #3 {
        n199 = Not Equal?(x=w474, y=w473) -> (x != y?=w472:bool)
        n200 = case shown="True" w472 {
          tunnel: w477 -> [_ w485]
          tunnel: w476 -> [_ w484]
          tunnel: [w478 w482] -> w475
          tunnel: w471 -> [w478 w479]
          frame #0 {
          }
          frame #1 {
            w480 = u16 1 items=["RAMP", "PAUSE", "MANUAL UP", "MANUAL DOWN", "ZERO"] ("Ramping Mode")
            n201 = call <userlib>:"Set Ramping Mode.vi"("error in"=w479, "Ramping Mode"=w480, "Communications Config"=w485) -> ("error out"=w483:T5)
            n202 = call <userlib>:"Set Ramping Mode.vi"("error in"=w483, "Ramping Mode"=w480, "Communications Config"=w484) -> ("error out"=w482:T5)
            n203 = local write "STATUS"("All Programmers are PAUSED. Set Ramping Mode to NEXT VECTOR to continue." ("STATUS")) -> ()
          }
        }
      }
      frame #4 {
        n204 = Not Equal?(x=w489, y=w491) -> (x != y?=w490:bool)
        n205 = case shown="False" w490 {
          tunnel: w494 -> [_ w503]
          tunnel: w493 -> [_ w502]
          tunnel: [w495 w498] -> w492
          tunnel: w488 -> [_ w501]
          tunnel: w487 -> [_ w500]
          tunnel: w486 -> [w495 w496]
          frame #0 {
          }
          frame #1 {
            w497 = u16 4 items=["RAMP", "PAUSE", "MANUAL UP", "MANUAL DOWN", "ZERO"] ("Ramping Mode")
            n206 = local write "STATUS"("Zeroing vector." ("STATUS")) -> ()
            n207 = call <userlib>:"Set Ramping Mode.vi"("error in"=w496, "Ramping Mode"=w497, "Communications Config"=w503) -> ("error out"=w506:T5)
            n208 = call <userlib>:"Set Ramping Mode.vi"("error in"=w506, "Ramping Mode"=w497, "Communications Config"=w502) -> ("error out"=w499:T5)
            n209 = call <userlib>:"Set Current Ramp Rate.vi"("Communications Config"=w503, "Ramp Rate (A/sec)"=w501, "error in"=w499) -> ("error out"=w504:T5)  [unwired: 2 in]
            n210 = call <userlib>:"Set Current Ramp Rate.vi"("Communications Config"=w502, "Ramp Rate (A/sec)"=w500, "error in"=w504) -> ("error out"=w498:T5)  [unwired: 2 in]
          }
        }
      }
    }
    n211 = local read "Continue Execution?"() -> (w247:bool)
    n212 = Wait Until Next ms Multiple(millisecond multiple=u32 100) -> ()  [unwired: 1 out]
  }
  n213 = case shown="0, Default" w29 {
    tunnel: w25 -> [w509 _ _]
    tunnel: w23 -> [w508 w512 w513]
    tunnel: [w507 w511 w513] -> w30
    tunnel: w24 -> [_ w510 _]
    frame #0 {
      n214 = call <userlib>:"430_TCP_Close.vi"("error in (no error)"=w508, "connection ID"=w509) -> ("error out"=w507:errorcluster)  [unwired: 1 out]
    }
    frame #1 {
      n215 = call <userlib>:"430_RS232_Close.vi"("error in (no error)"=w512, "VISA resource name"=w510) -> ("error out"=w511:errorcluster)  [unwired: 1 in]
    }
    frame #2 {
    }
  }
  n216 = case shown="0, Default" w28 {
    tunnel: w27 -> [w516 _ _]
    tunnel: w30 -> [w515 w519 w520]
    tunnel: [w514 w518 w520] -> w20
    tunnel: w26 -> [_ w517 _]
    frame #0 {
      n217 = call <userlib>:"430_TCP_Close.vi"("error in (no error)"=w515, "connection ID"=w516) -> ("error out"=w514:errorcluster)  [unwired: 1 out]
    }
    frame #1 {
      n218 = call <userlib>:"430_RS232_Close.vi"("error in (no error)"=w519, "VISA resource name"=w517) -> ("error out"=w518:errorcluster)  [unwired: 1 in]
    }
    frame #2 {
    }
  }
  "error out" <- w20
  n219 = local read "Magnetic Field Units"() -> (w47:u16)
  n220 = local read "Coordinate System"() -> (w48:u16)
  n221 = while {
    tunnel: "Starting index" -> [w528]
    tunnel: w22 -> [w534]
    tunnel: w21 -> [w535]
    tunnel: w47 -> [w536]
    tunnel: w48 -> [w537]
    tunnel: w45 -> [w540]
    tunnel: "Max Ramp Rate - Y Axis (A/s)" -> [w524]
    tunnel: "Max Ramp Rate - Z Axis (A/s)" -> [w523]
    tunnel: "Magnitude Limit (kG)" -> [w525]
    tunnel: "User defined Ramp Rate (T/min)" -> [w522]
    tunnel: "User defined Ramp Rate (T/min)" -> [w521]
    i -> [w527]
    stop <- w529 continue-if-true
    n222 = local read "Field Values"() -> (w531:string[][])
    n223 = Add(x=w528, y=w527) -> (x+y=w526:i32)
    n224 = while "Wait for NEXT VECTOR setting by operator." {
      tunnel: [w544] -> w539
      tunnel: w540 -> [w544]
      stop <- w545 continue-if-true
      w543 = u16 0 items=["NEXT VECTOR", "RAMPING", "HOLDING", "PAUSE", "ZERO"] ("Ramping Control")
      n225 = local read "Ramping Control"() -> (w546:u16)
      n226 = Not Equal?(x=w543, y=w546) -> (x != y?=w545:bool)
    }
    n227 = stacked-sequence {
      tunnel: w526 -> [w548 _ w554 _]
      frame #0 {
        (unwired) -2
        n228 = Subtract(x=w548, y=2) -> (x-y=w551:i32)
        n229 = Bundle(w551, -2) -> (w549:cluster{i32, i32})  [unwired: 1 in]
        n230 = property on="Field Values" class="Tbl (strict)"("Active Cell:Active Cell"=w549) -> ()  [unwired: 2 in, 2 out]
      }
      frame #1 {
        n231 = local read "Normal color"() -> (w552:u32)
        n232 = property on="Field Values" class="Tbl (strict)"("Active Cell:Cell Background Color"=w552) -> ()  [unwired: 2 in, 2 out]
      }
      frame #2 {
        n233 = Decrement(x=w554) -> (x-1=w553:i32)
        n234 = Bundle(w553, -2) -> (w556:cluster{i32, i32})  [unwired: 1 in]
        n235 = property on="Field Values" class="Tbl (strict)"("Active Cell:Active Cell"=w556) -> ()  [unwired: 2 in, 2 out]
      }
      frame #3 {
        n236 = property on="Field Values" class="Tbl (strict)"("Active Cell:Cell Background Color"="Highlight color") -> ()  [unwired: 2 in, 2 out]
      }
    }
    n237 = Index Array(array=w531, index (row)=w526) -> (element=w538:string[])  [unwired: 1 in]
    n238 = local write "Starting index"(w526) -> ()
    n239 = Add(x=1, y=w526) -> (x+y=w541:i32)
    n240 = Number To Decimal String(number=w541) -> (decimal integer string=w530:string)  [unwired: 1 in]
    n241 = stacked-sequence {
      tunnel: [_ w582] -> w532
      tunnel: [_ w581] -> w533
      tunnel: w539 -> [_ w577]
      tunnel: w538 -> [_ w576]
      tunnel: w537 -> [_ w575]
      tunnel: w536 -> [_ w574]
      tunnel: w535 -> [_ w573]
      tunnel: w534 -> [_ w572]
      tunnel: w530 -> [_ w571]
      tunnel: w525 -> [_ w569]
      tunnel: w524 -> [_ w568]
      tunnel: w523 -> [_ w563]
      tunnel: w522 -> [_ w567]
      tunnel: w521 -> [_ w566]
      frame #0 {
        w561 = u16 1 items=["NEXT VECTOR", "RAMPING", "HOLDING", "PAUSE", "ZERO"] ("Ramping Control")
        n242 = local write "Ramping Control"(w561) -> ()
      }
      frame #1 {
        n243 = call <userlib>:"Set 2D Next Vector_entwurf.vi"("Coordinate System"=w575, "Magnetic Field Units"=w574, 3:"User defined Ramp Rate (T/min)"=w566, "Magnitude Limit (kG)"=w569, "Y-Axis Communications Config"=w573, "Input Vector"=w576, "Z-Axis Communications Config"=w572, 10:"User defined Ramp Rate (T/min)"=w567, "Max Ramp Rate - Y Axis (A/s)"=w568, "error in"=w577, "Max Ramp Rate - Z Axis (A/s)"=w563) -> ("Y-Axis Ramp Rate (T/min)"=→"Current Ramp Rate Y (T/min)":dbl, "Within Limits?"=w582:bool, "Ramp Rate along Vector (T/min)"=→"Ramp Rate along Vector (T/min)":dbl, "Z-Axis Ramp Rate (T/min)"=→"Current Ramp Rate Z (T/min)":dbl, "All Instruments Responded?"=w581:bool, "error out"=w570:T5)  [unwired: 3 in]
        n244 = Concatenate Strings("Ramping to field vector " ("STATUS"), w571, "..." ("STATUS")) -> (w578:string)
        n245 = local write "error in"(w570) -> ()
        n246 = local write "STATUS"(w578) -> ()
      }
    }
    n247 = case shown="True" w532 {
      tunnel: w533 -> [_ w559]
      frame #0 {
        n248 = local write "STATUS"("Vector magnitude limt or maximum coil current exceeded. Vector ignored. VI halted." ("STATUS")) -> ()
      }
      frame #1 {
        n249 = case shown="True" w559 {
          frame #0 {
            n250 = local write "STATUS"("Not all programmers responded. VI halted." ("STATUS")) -> ()
          }
          frame #1 {
          }
        }
      }
    }
    n251 = Compound Arithmetic op=AND(w533, w532) -> (w529:bool)
    n252 = local write "Continue Execution?"(w529) -> ()
  }
